vi "test wrap and unwrap.vi"() -> ()   [LabVIEW 2013, in "TBM Tests.lvlib"]
uses:
  TBM Tests.lvlib
  root configuration/TBM configuration.lvclass
panel:
  out "OK if not found":bool
  out "array":T1(array[cluster])
  out "ok":bool
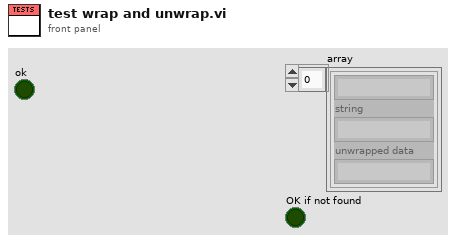
[diagram p1: front panel]
types:
  T1 = cluster{string, "string":string, "unwrapped data":string}[]
  T2 = cluster{string, "string":string, "unwrapped data":string}
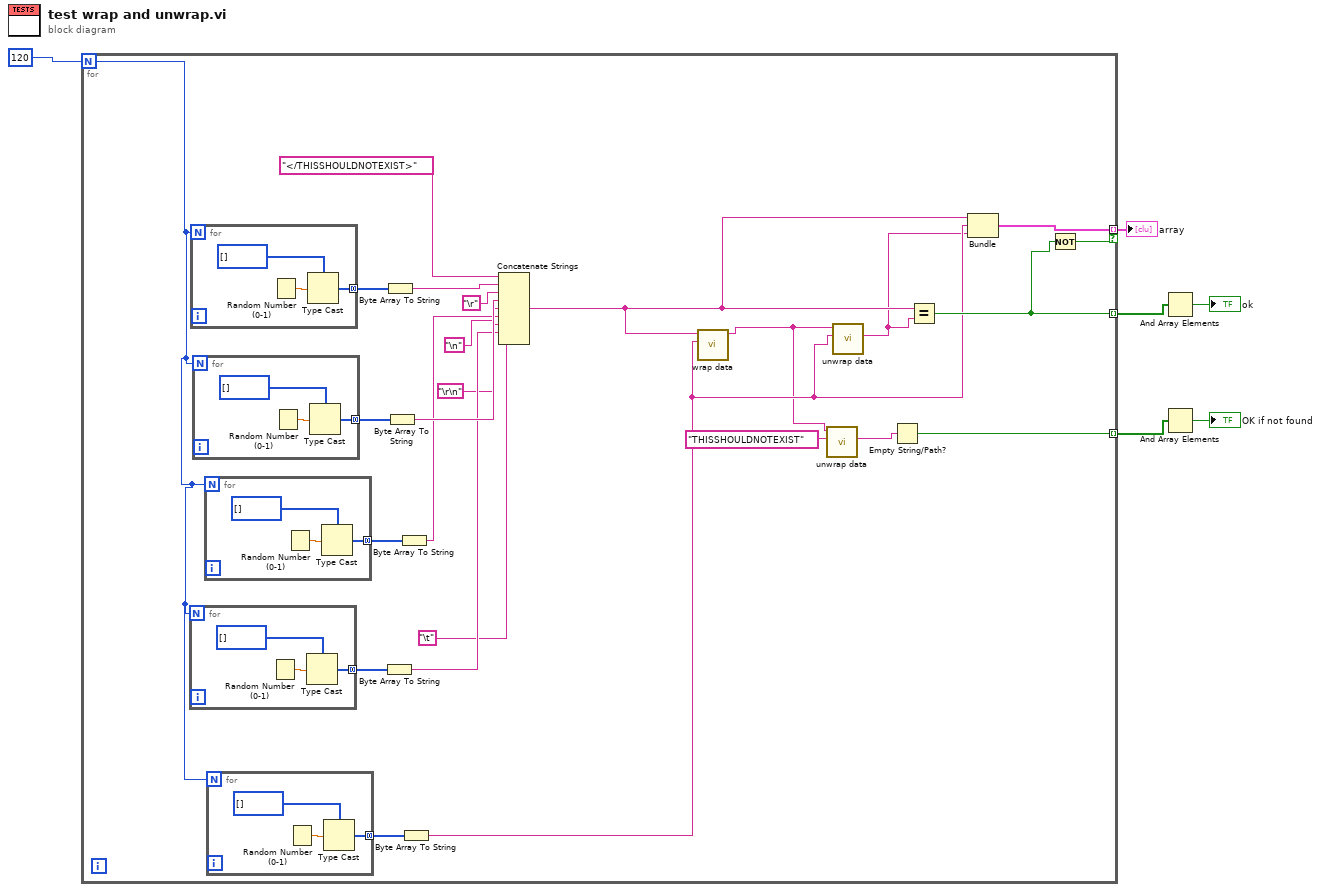
[diagram p0: block diagram]
diagram:
  n1 = for {
    N: 120 -> [w18]
    tunnel: [w15] -> w5 mode=indexing
    tunnel: [w16] -> w3 mode=indexing if=w14
    tunnel: [w8] -> w2 mode=indexing
    n2 = for {
      N: w18 -> [_]
      tunnel: [w35] -> w28 mode=concatenating
      n3 = Random Number (0-1)() -> (number: 0 to 1=w37:dbl)
      n4 = Type Cast(type=u8[] [], x=w37) -> (*(type *) &x=w35:u8[])
    }
    n5 = for {
      N: w18 -> [_]
      tunnel: [w44] -> w31 mode=concatenating
      n6 = Random Number (0-1)() -> (number: 0 to 1=w46:dbl)
      n7 = Type Cast(type=u8[] [], x=w46) -> (*(type *) &x=w44:u8[])
    }
    n8 = for {
      N: w18 -> [_]
      tunnel: [w41] -> w30 mode=concatenating
      n9 = Random Number (0-1)() -> (number: 0 to 1=w43:dbl)
      n10 = Type Cast(type=u8[] [], x=w43) -> (*(type *) &x=w41:u8[])
    }
    n11 = for {
      N: w18 -> [_]
      tunnel: [w38] -> w29 mode=concatenating
      n12 = Random Number (0-1)() -> (number: 0 to 1=w40:dbl)
      n13 = Type Cast(type=u8[] [], x=w40) -> (*(type *) &x=w38:u8[])
    }
    n14 = for {
      N: w18 -> [_]
      tunnel: [w32] -> w19 mode=concatenating
      n15 = Random Number (0-1)() -> (number: 0 to 1=w34:dbl)
      n16 = Type Cast(type=u8[] [], x=w34) -> (*(type *) &x=w32:u8[])
    }
    n17 = Byte Array To String(unsigned byte array=w28) -> (string=w24:string)
    n18 = Byte Array To String(unsigned byte array=w31) -> (string=w27:string)
    n19 = Byte Array To String(unsigned byte array=w30) -> (string=w26:string)
    n20 = Byte Array To String(unsigned byte array=w29) -> (string=w25:string)
    n21 = Byte Array To String(unsigned byte array=w19) -> (string=w13:string)
    n22 = Concatenate Strings("</THISSHOULDNOTEXIST>" ("string"), w27, "\r", w26, "\n", w25, "\r\n", w24, "\t") -> (w17:string)
    n23 = call "wrap data.vi"("identifier"=w13, "data to wrap"=w17) -> ("wrapped data"=w11:string)  [unwired: 9 in]
    n24 = call "unwrap data.vi"("identifier"="THISSHOULDNOTEXIST", "data to unwrap"=w11) -> ("unwrapped data"=w9:string)  [unwired: 8 in, 1 out]
    n25 = call "unwrap data.vi"("identifier"=w13, "data to unwrap"=w11) -> ("unwrapped data"=w12:string)  [unwired: 8 in, 1 out]
    n26 = Empty String/Path?(string/path=w9) -> (empty?=w8:bool)
    n27 = Equal?(x=w17, y=w12) -> (x = y?=w15:bool)
    n28 = Bundle(w17, "string"=w13, "unwrapped data"=w12) -> (w16:T2)  [unwired: 1 in]
    n29 = Not(x=w15) -> (.not. x?=w14:bool)
  }
  "array" <- w3
  n30 = And Array Elements(Boolean array=w5) -> (logical AND=→"ok":bool)
  n31 = And Array Elements(Boolean array=w2) -> (logical AND=→"OK if not found":bool)
